vi "Init_graphe.vi"() -> ()   [LabVIEW 2013]
uses:
  <vilib>/Utility/miscctls.llb/LVRowAndColumnTypeDef.ctl
  <vilib>/Utility/miscctls.llb/LVRowAndColumnUnsignedTypeDef.ctl
  <vilib>/Utility/file.llb/Read From Spreadsheet File (string).vi
panel:
  out "Nb lignes":i32
  in  "N° colonne Y":i8=2 min=1
  in  "N° colonne X":i8=1 min=1
  in  "Nbre lignes entête":i8=2 min=1
  in  "Bouton Aide":bool
  in  "Quit":bool
  in  "Fichier données brutes":path
  out "Colonne données brutes":string="0"
  out "Noms variables":string[](array[string])
  out "Séparateur fichier brute":string
  in  "Valider":bool
  in  "Séparateur":u16(ring)=5 items=["", ",", ";", ".", "Tab", "Espace", ":"]
  out "Table":string[][](table)
  # "Sélectionner la 1ère cellule\ndes noms de variables"
  # "Facultatif : \nSélectionner la dernière cellule des noms de variables  en appuyant sur la touche CTRL"
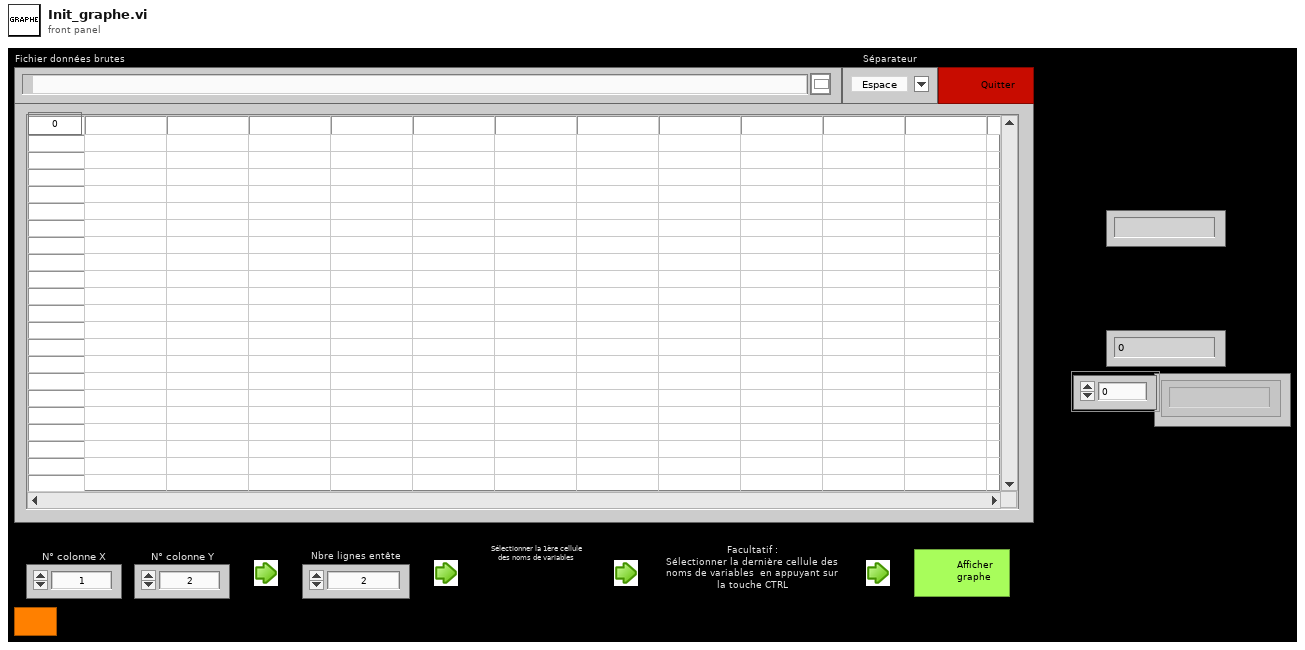
[diagram p1: front panel]
types:
  T1 = typedef "LVRowAndColumnTypeDef.ctl" = cluster{"Row":i32, "Column":i32}
  T2 = typedef "LVRowAndColumnUnsignedTypeDef.ctl" = cluster{"Row":u32, "Column":u32}
  T3 = typedef "excel Object Reference.ctl" = refnum<k1>
  T4 = cluster{"Shift":bool, "Ctrl":bool, "Alt":bool, "Cmd":bool, "Opt":bool}
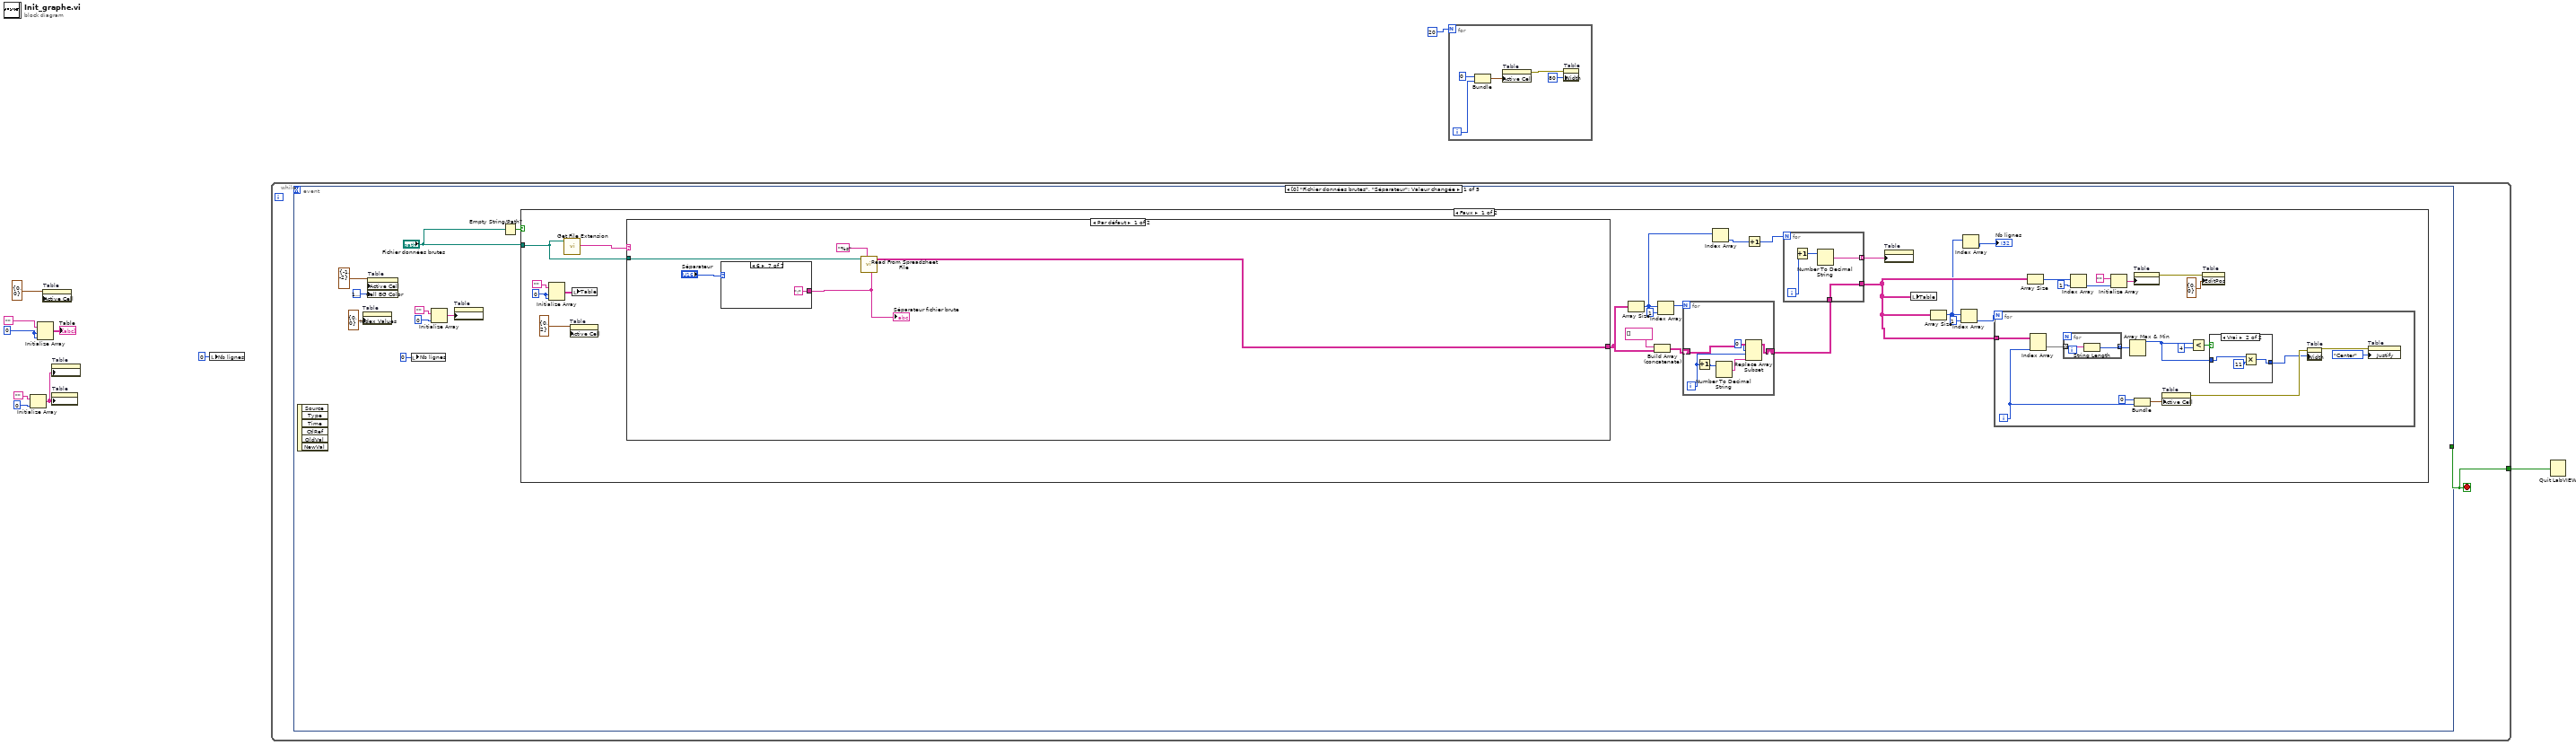
[diagram p0: block diagram]
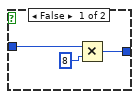
[diagram p2: hidden frame]
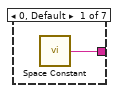
[diagram p3: hidden frame]
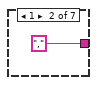
[diagram p4: hidden frame]
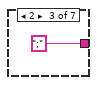
[diagram p5: hidden frame]
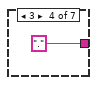
[diagram p6: hidden frame]
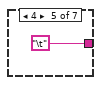
[diagram p7: hidden frame]
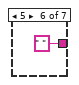
[diagram p8: hidden frame]
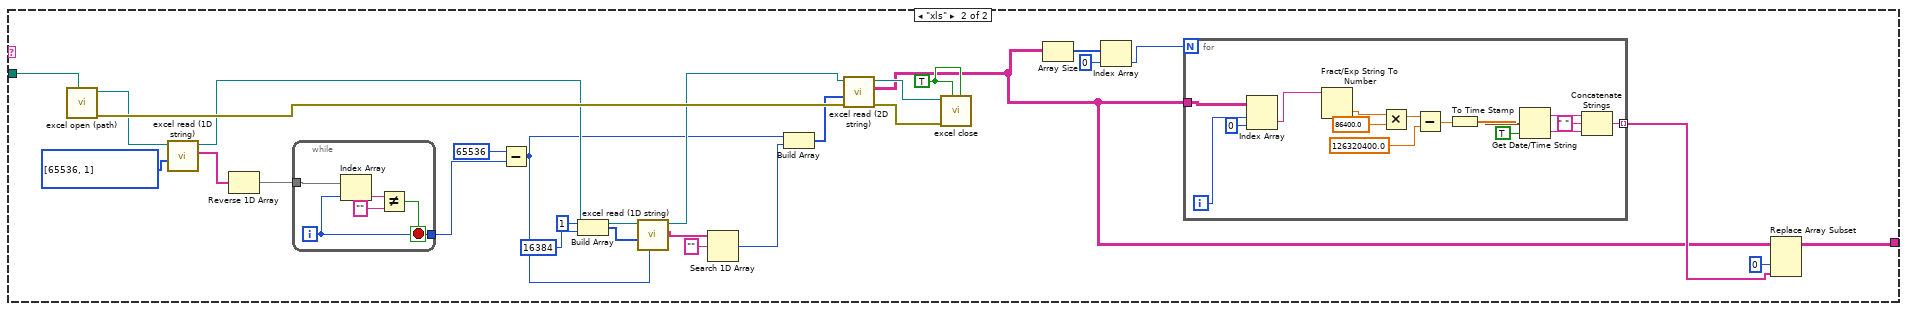
[diagram p9: hidden frame]
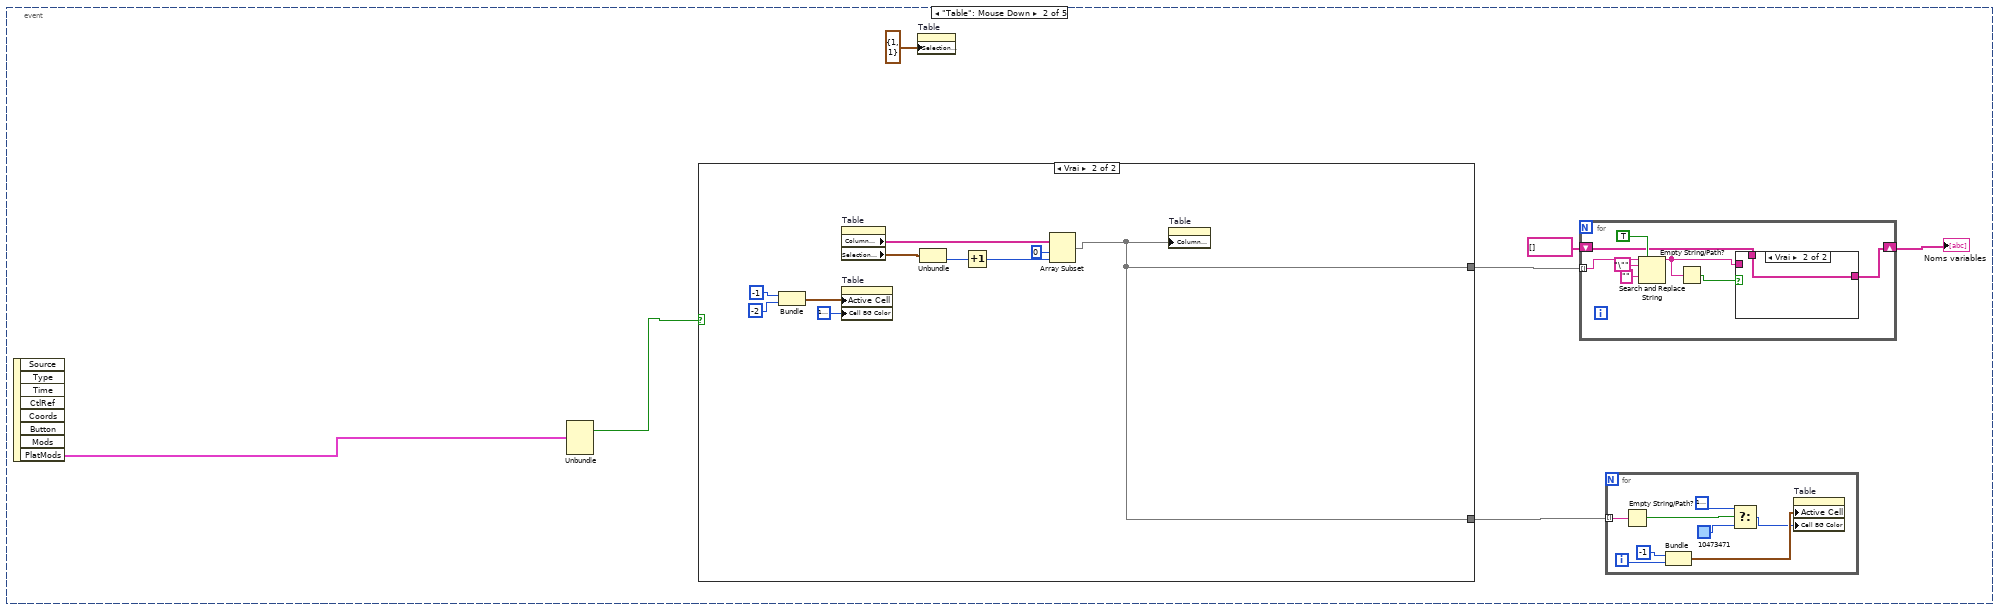
[diagram p11: hidden frame]
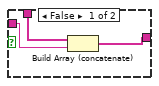
[diagram p12: hidden frame]
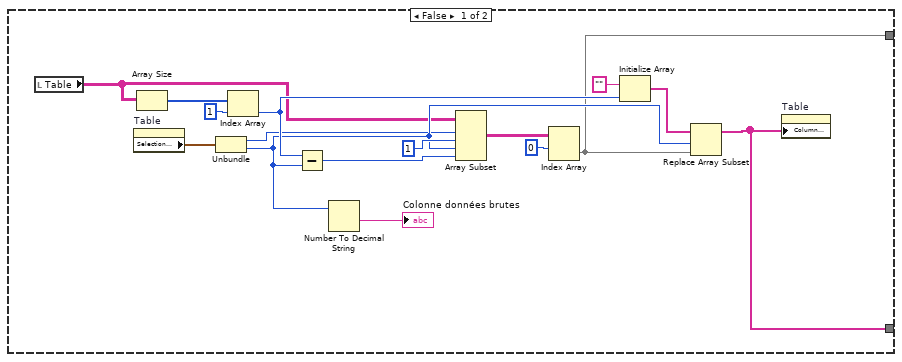
[diagram p13: hidden frame]
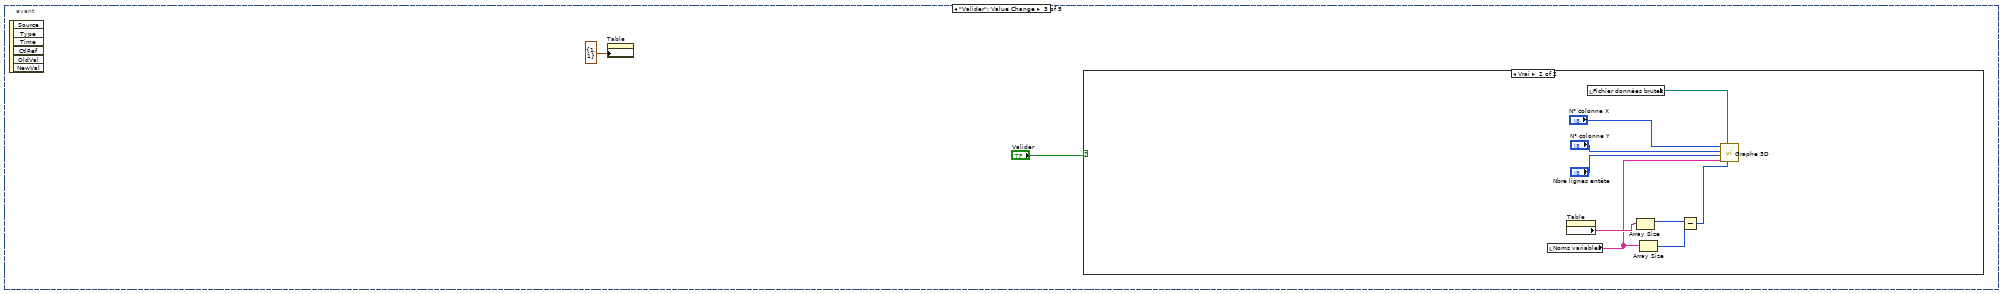
[diagram p14: hidden frame]
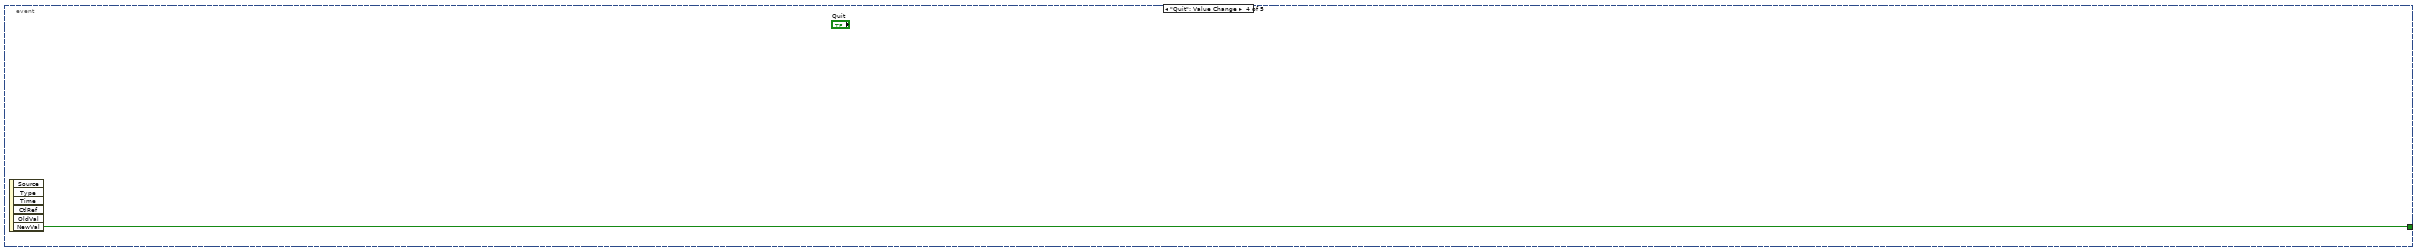
[diagram p16: hidden frame]
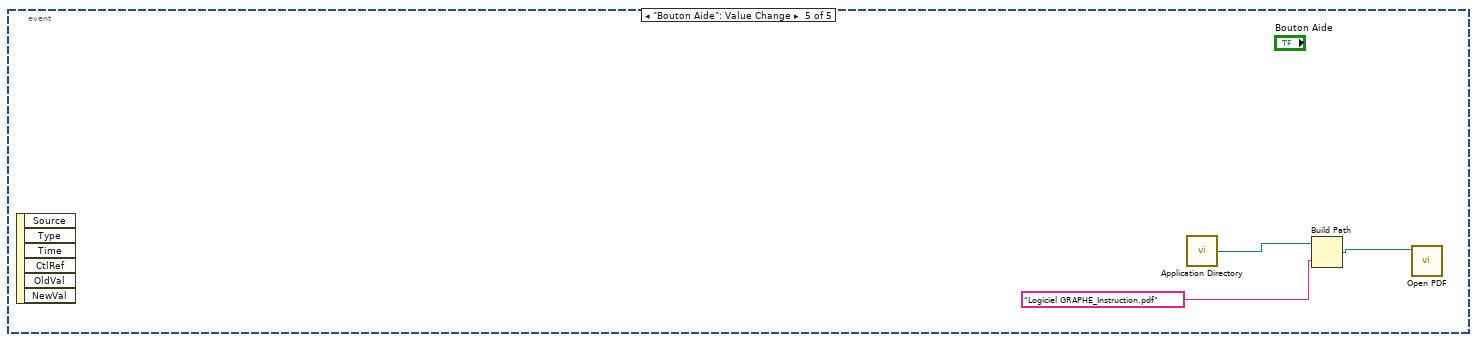
[diagram p17: hidden frame]
diagram:
  w5 = 0 ("taille de la dimension")
  n1 = Initialize Array("", 0 ("taille de la dimension")) -> (w10:string[])
  n2 = Initialize Array("", w5, w5) -> (→"Table":string[][])
  n3 = property on="Table" class="Tbl (strict)"("Active Cell"=T1 {"Row"=0, "Column"=0} ("Cellule active:Cellule active")) -> ()  [unwired: 2 in, 2 out]
  n4 = property on="Table" class="Tbl (strict)"("Row Headers[]"=w10) -> ()  [unwired: 2 in, 2 out]
  n5 = property on="Table" class="Tbl (strict)"("Column Headers[]"=w10) -> ()  [unwired: 2 in, 2 out]
  n6 = local write "Nb lignes"(0 ("Nb lignes")) -> ()
  n7 = while {
    tunnel: [w11] -> w3
    stop <- w11 stop-if-true
    n8 = event shown="[0] \"Fichier données brutes\", \"Séparateur\": Valeur changée" {
      selector: _ -> [_ _ _ _ _]
      dyn-events: _ -> [_ _ _ _ _]
      timeout: _ -> [_ _ _ _ _]
      tunnel: [_ _ _ w204 _] -> w11
      event "Fichier données brutes", "Séparateur": Value Change {
        n9 = event-data() -> ()  [unwired: 1 in, 6 out]
        n10 = property on="Table" class="Tbl (strict)"("Index Values"=T2 {"Row"=0, "Column"=0} ("Valeurs d'indice")) -> ()  [unwired: 2 in, 2 out]
        n11 = property on="Table" class="Tbl (strict)"("Active Cell"=T1 {"Row"=-1, "Column"=-2} ("Cellule active:Cellule active"), "Cell BG Color"=u32 16777225) -> ()  [unwired: 2 in, 2 out]
        n12 = local write "Nb lignes"(0 ("Nb lignes")) -> ()
        n13 = Initialize Array("", 0 ("taille de la dimension")) -> (w15:string[])
        n14 = property on="Table" class="Tbl (strict)"("Row Headers[]"=w15) -> ()  [unwired: 2 in, 2 out]
        n15 = Empty String/Path?(string/path="Fichier données brutes") -> (empty?=w20:bool)
        n16 = case shown="Faux" w20 {
          tunnel: "Fichier données brutes" -> [w41 _]
          frame False {
            w37 = 0 ("taille de la dimension")
            n17 = Initialize Array("", w37, w37) -> (w35:string[][])
            n18 = call <vilib>:"Get File Extension.vi"("file"=w41) -> ("lowercase file extension"=w40:string)  [unwired: 7 in, 3 out]
            n19 = property on="Table" class="Tbl (strict)"("Active Cell"=T1 {"Row"=0, "Column"=2} ("Cellule active:Cellule active")) -> ()  [unwired: 2 in, 2 out]
            n20 = local write "Table"(w35) -> ()
            n21 = case shown="Par défaut" w40 {
              tunnel: w41 -> [w83 w119]
              tunnel: [w82 w92] -> w30
              frame Default {
                n22 = case shown="6" "Séparateur" {
                  tunnel: [w85 "," ";" "." "\t" " " ("String") ":" ("String")] -> w80
                  frame 0, Default {
                    n23 = call <vilib>:"Space Constant.vi"() -> ("String"=w85:string)
                  }
                  frame 1 {
                  }
                  frame 2 {
                  }
                  frame 3 {
                  }
                  frame 4 {
                  }
                  frame 5 {
                  }
                  frame 6 {
                  }
                }
                "Séparateur fichier brute" <- w80
                n24 = call-poly <vilib>:"Read From Spreadsheet File.vi"("delimiter (\\t)"=w80, "format (%s)"="%s", "file path (dialog if empty)"=w83) -> ("all rows"=w82:string[][])  [unwired: 4 in, 4 out]
              }
              frame "xls" {
                w115 = TRUE ("Override closing behavior")
                n25 = call <userlib>:"excel open (path).vi"("workbook path"=w119) -> ("error out"=w116:errorcluster, "reference"=w114:T3)  [unwired: 9 in]
                n26 = call <userlib>:"excel read (1D string).vi"("array size\n  - #rows\n  - #columns"=i32[] [65536, 1] ("array size\n  - #rows\n  - #columns"), "reference"=w114) -> ("1D String Array"=w112:string[], "duplicate reference"=w105:T3)  [unwired: 7 in, 1 out]
                n27 = Reverse 1D Array(array=w112) -> (reversed array=w110:string[])
                n28 = while {
                  tunnel: w110 -> [w139]
                  tunnel: [w135] -> w109
                  i -> [w135]
                  stop <- w136 stop-if-true
                  n29 = Index Array(array=w139, index=w135) -> (element=w138:string)
                  n30 = Not Equal?(x=w138, y="") -> (x != y?=w136:bool)
                }
                n31 = Subtract(x=65536, y=w109) -> (x-y=w102:i32)
                n32 = Build Array(1 ("élément"), 16384 ("élément")) -> (w106:i32[])
                n33 = call <userlib>:"excel read (1D string).vi"("Row"=w102, "array size\n  - #rows\n  - #columns"=w106, "reference"=w105) -> ("1D String Array"=w101:string[], "duplicate reference"=w104:T3)  [unwired: 6 in, 1 out]
                n34 = Search 1D Array(1D array=w101, element="" ("élément")) -> (index of element=w99:i32)  [unwired: 1 in]
                n35 = Build Array(w102, w99) -> (w111:i32[])
                n36 = call <userlib>:"excel read (2D string).vi"("error in (no error)"=w116, "array size\n  - #rows\n  - #columns"=w111, "reference"=w104) -> ("error out"=w117:errorcluster, "2D String Array"=w93:string[][], "duplicate reference"=w118:T3)  [unwired: 6 in]
                n37 = call <userlib>:"excel close.vi"("Close"=w115, "Override closing behavior"=w115, "error in (no error)"=w117, "reference"=w118) -> ()  [unwired: 7 in, 1 out]
                n38 = Array Size(array=w93) -> (size(s)=w95:i32[])
                n39 = Index Array(array=w95, index=0 ("indice")) -> (element=w96:i32)
                n40 = for {
                  N: w96 -> [_]
                  tunnel: w93 -> [w134]
                  tunnel: [w120] -> w98 mode=indexing
                  i -> [w133]
                  n41 = Index Array(array=w134, index (row)=w133, index (col)=0 ("indice désactivé (col)")) -> (element=w121:string)
                  n42 = Fract/Exp String To Number(string=w121) -> (number=w131:dbl)  [unwired: 3 in, 1 out]
                  n43 = Multiply(x=w131, y=86400.0) -> (x*y=w129:dbl)
                  n44 = Subtract(x=w129, y=126320400.0) -> (x-y=w127:dbl)
                  n45 = To Time Stamp(1:w127) -> (0:w126:timestamp)
                  n46 = Get Date/Time String(seconds (now)=w126, want seconds? (F)=TRUE ("secondes ? (F)")) -> (date string=w124:string, time string=w122:string)  [unwired: 1 in]
                  n47 = Concatenate Strings(w124, " " ("chaîne"), w122) -> (w120:string)
                }
                n48 = Replace Array Subset(array=w93, new element=w98, index (col)=0 ("indice désactivé (col)")) -> (w92:string[][])  [unwired: 1 in]
              }
            }
            n49 = Array Size(array=w30) -> (size(s)=w27:i32[])
            n50 = Build Array (concatenate)(string[] [] ("élément"), w30) -> (w34:string[][])
            n51 = Index Array(array=w27, index=1 ("indice")) -> (element=w32:i32)
            n52 = for {
              N: w32 -> [_]
              shift-right: [w58] -> w26
              shift-left: w34 -> [w57]
              i -> [w54]
              n53 = Increment(x=w54) -> (x+1=w56:i32)
              n54 = Number To Decimal String(number=w56) -> (decimal integer string=w53:string)  [unwired: 1 in]
              n55 = Replace Array Subset(array=w57, new element=w53, index (row)=0 ("indice désactivé (ligne)"), index (col)=w54) -> (w58:string[][])
            }
            n56 = Index Array(array=w27) -> (element=w28:i32)  [unwired: 1 in]
            n57 = Increment(x=w28) -> (x+1=w23:i32)
            n58 = for {
              N: w23 -> [_]
              tunnel: w26 -> [w52]
              tunnel: [w52] -> w25
              tunnel: [w49] -> w24 mode=indexing
              i -> [w51]
              n59 = Increment(x=w51) -> (x+1=w50:i32)
              n60 = Number To Decimal String(number=w50) -> (decimal integer string=w49:string)  [unwired: 1 in]
            }
            n61 = property on="Table" class="Tbl (strict)"("Row Headers[]"=w24) -> ()  [unwired: 2 in, 2 out]
            n62 = local write "Table"(w25) -> ()
            n63 = Array Size(array=w25) -> (size(s)=w21:i32[])
            n64 = Index Array(array=w21, index=1 ("indice")) -> (element=w39:i32)
            n65 = Index Array(array=w21) -> (element=→"Nb lignes":i32)  [unwired: 1 in]
            n66 = for {
              N: w39 -> [_]
              tunnel: w25 -> [w71]
              i -> [w66]
              n67 = Index Array(array=w71, index (col)=w66) -> (element=w70:string[])  [unwired: 1 in]
              n68 = for {
                tunnel: w70 -> [w79] mode=indexing
                tunnel: [w78] -> w69 mode=indexing
                n69 = String Length(string=w79) -> (length=w78:i32)
              }
              n70 = Array Max & Min(array=w69) -> (max value=w60:i32)  [unwired: 3 out]
              n71 = Bundle(0, w66) -> (w68:cluster{i32, i32})  [unwired: 1 in]
              n72 = property on="Table" class="Tbl (strict)"("Active Cell"=w68) -> (error out=w67:errorcluster)  [unwired: 2 in, 1 out]
              n73 = Less?(x=w60, y=4) -> (x < y?=w61:bool)
              n74 = case shown="Vrai" w61 {
                tunnel: [w74 w75] -> w59
                tunnel: w60 -> [w72 w76]
                frame False {
                  n75 = Multiply(x=w72, y=8) -> (x*y=w74:i32)
                }
                frame True {
                  n76 = Multiply(x=w76, y=11) -> (x*y=w75:i32)
                }
              }
              n77 = property on="Table" class="Tbl (strict)"(error in=w67, "Width"=w59) -> (error out=w64:errorcluster)  [unwired: 1 in, 1 out]
              n78 = property on="Table" class="Tbl (strict)"(error in=w64, "Justify"=enum16{"Left", "Center", "Right"}."Center" ("Cellule active:Justification de la cellule")) -> ()  [unwired: 1 in, 2 out]
            }
            n79 = Array Size(array=w25) -> (size(s)=w48:i32[])
            n80 = Index Array(array=w48, index=1 ("indice")) -> (element=w44:i32)
            n81 = Initialize Array("", w44) -> (w45:string[])
            n82 = property on="Table" class="Tbl (strict)"("Column Headers[]"=w45) -> (error out=w42:errorcluster)  [unwired: 2 in, 1 out]
            n83 = property on="Table" class="Tbl (strict)"(error in=w42, "EditPos"=T1 {"Row"=0, "Column"=0} ("Cellule active:Cellule active")) -> ()  [unwired: 1 in, 2 out]
          }
          frame True {
          }
        }
      }
      event "Table": Mouse Down {
        n84 = event-data() -> ("PlatMods"=w145:T4)  [unwired: 1 in, 7 out]
        n85 = Unbundle(w145) -> ("Ctrl"=w144:bool)  [unwired: 4 out]
        n86 = case shown="Vrai" w144 {
          tunnel: [w170 w189] -> w141
          tunnel: [w168 w189] -> w140
          frame False {
            n87 = local read "Table"() -> (w167:string[][])
            n88 = property on="Table" class="Tbl (strict)"() -> ("Selection Start"=w169:T1)  [unwired: 2 in, 2 out]
            n89 = Array Size(array=w167) -> (size(s)=w180:i32[])
            n90 = Unbundle(w169) -> ("Row"=w171:i32, "Column"=w173:i32)
            n91 = Index Array(array=w180, index=1 ("indice")) -> (element=w174:i32)
            n92 = Subtract(x=w174, y=w173) -> (x-y=w178:i32)
            n93 = Number To Decimal String(number=w173) -> (decimal integer string=→"Colonne données brutes":string)  [unwired: 1 in]
            n94 = Array Subset(array=w167, index (row)=w171, length (row)=1 ("longueur"), index (col)=w173, length (col)=w178) -> (w181:string[][])
            n95 = Index Array(array=w181, index (row)=0 ("indice (ligne)")) -> (element=w170:string[])  [unwired: 1 in]
            n96 = Initialize Array("", w174) -> (w176:string[])
            n97 = Replace Array Subset(array=w176, new element=w170, index=w173) -> (w168:string[])
            n98 = property on="Table" class="Tbl (strict)"("Column Headers[]"=w168) -> ()  [unwired: 2 in, 2 out]
          }
          frame True {
            n99 = Bundle(-1, -2) -> (w186:cluster{i32, i32})  [unwired: 1 in]
            n100 = property on="Table" class="Tbl (strict)"() -> ("Column Headers[]"=w188:string[], "Selection Start"=w183:T1)  [unwired: 2 in, 2 out]
            n101 = property on="Table" class="Tbl (strict)"("Active Cell"=w186, "Cell BG Color"=u32 16777225) -> ()  [unwired: 2 in, 2 out]
            n102 = Unbundle(w183) -> ("Column"=w190:i32)  [unwired: 1 out]
            n103 = Increment(x=w190) -> (x+1=w192:i32)
            n104 = Array Subset(array=w188, index=0 ("indice"), length=w192) -> (w189:string[])
            n105 = property on="Table" class="Tbl (strict)"("Column Headers[]"=w189) -> ()  [unwired: 2 in, 2 out]
          }
        }
        n106 = property on="Table" class="Tbl (strict)"("Selection Size"=T1 {"Row"=1, "Column"=1} ("Taille de sélection")) -> ()  [unwired: 2 in, 2 out]
        n107 = for {
          tunnel: w141 -> [w155] mode=indexing
          shift-right: [w157] -> w143
          shift-left: string[] [] -> [w158]
          n108 = Search and Replace String(replace all?=TRUE ("tout remplacer ? (F)"), input string=w155, search string="\"" ("chaîne recherchée"), replace string="" ("chaîne de remplacement (\"\")")) -> (result string=w156:string)  [unwired: 4 in, 3 out]
          n109 = Empty String/Path?(string/path=w156) -> (empty?=w159:bool)
          n110 = case shown="Vrai" w159 {
            tunnel: w158 -> [w165 w166]
            tunnel: [w163 w166] -> w157
            tunnel: w156 -> [w164 _]
            frame False {
              n111 = Build Array (concatenate)(w165, w164) -> (w163:string[])
            }
            frame True {
            }
          }
        }
        "Noms variables" <- w143
        n112 = for {
          tunnel: w140 -> [w154] mode=indexing
          i -> [w152]
          n113 = Empty String/Path?(string/path=w154) -> (empty?=w150:bool)
          n114 = Bundle(-1, w152) -> (w151:cluster{i32, i32})  [unwired: 1 in]
          n115 = Select(t=u32 16777225, s=w150, f=u32 10473471) -> (s? t:f=w147:u32)
          n116 = property on="Table" class="Tbl (strict)"("Active Cell"=w151, "Cell BG Color"=w147) -> ()  [unwired: 2 in, 2 out]
        }
      }
      event "Valider": Value Change {
        n117 = event-data() -> ()  [unwired: 1 in, 6 out]
        n118 = property on="Table" class="Tbl (strict)"("Selection Size"=T1 {"Row"=1, "Column"=1} ("Taille de sélection")) -> ()  [unwired: 2 in, 2 out]
        n119 = case shown="Vrai" "Valider" {
          frame False {
          }
          frame True {
            n120 = local read "Noms variables"() -> (w196:string[])
            n121 = property on="Table" class="Tbl (strict)"() -> ("Column Headers[]"=w199:string[])  [unwired: 2 in, 2 out]
            n122 = local read "Fichier données brutes"() -> (w200:path)
            n123 = Array Size(array=w199) -> (size(s)=w198:i32)
            n124 = Array Size(array=w196) -> (size(s)=w195:i32)
            n125 = Subtract(x=w198, y=w195) -> (x-y=w197:i32)
            n126 = call "Graphe 3D.vi"("Nbre colonnes"=w197, "file path (dialog if empty)"=w200, "Paramètres axe Z"=w196, "Nbre lignes entête"="Nbre lignes entête", "N° colonne Y"="N° colonne Y", "N° colonne X"="N° colonne X") -> ()  [unwired: 4 in]
          }
        }
      }
      event "Quit": Value Change {
        n127 = event-data() -> ("NewVal"=w204:bool)  [unwired: 1 in, 5 out]
      }
      event "Bouton Aide": Value Change {
        n128 = event-data() -> ()  [unwired: 1 in, 6 out]
        n129 = call <vilib>:"Application Directory.vi"() -> ("Application Directory"=w206:path)
        n130 = Build Path(base path=w206, name or relative path="Logiciel GRAPHE_Instruction.pdf" ("standard input")) -> (appended path=w205:path)
        n131 = call "Open PDF.vi"("Path"=w205) -> ()  [unwired: 5 in, 2 out]
      }
    }
  }
  n132 = for {
    N: 20 -> [_]
    i -> [w210]
    n133 = Bundle(0, w210) -> (w211:cluster{i32, i32})  [unwired: 1 in]
    n134 = property on="Table" class="Tbl (strict)"("Active Cell"=w211) -> (error out=w208:errorcluster)  [unwired: 2 in, 1 out]
    n135 = property on="Table" class="Tbl (strict)"(error in=w208, "Width"=u32 80 ("Cellule active:Taille de la cellule:Largeur")) -> ()  [unwired: 1 in, 2 out]
  }
  n136 = Quit LabVIEW(quit? (T)=w3) -> ()
